vi "Flat sequence in LabVIEW.vi"() -> ()   [LabVIEW 2026]
panel:
  out "MULTIPLY":dbl
  out "MINUS":dbl
  out "SUM":dbl
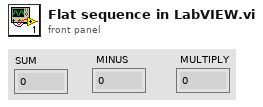
[diagram p1: front panel]
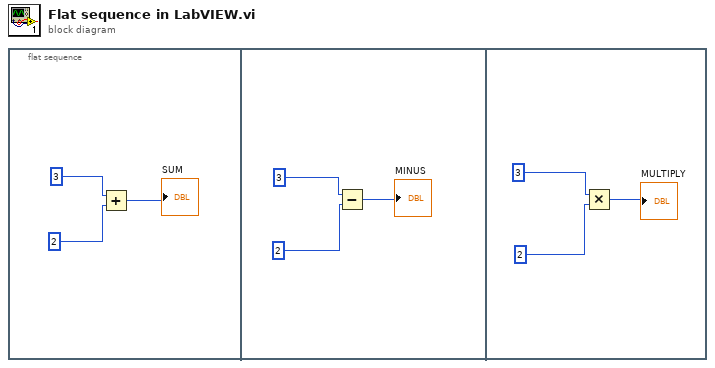
[diagram p0: block diagram]
diagram:
  n1 = flat-sequence {
    frame #0 {
      n2 = Add(x=3, y=2) -> (x+y=→"SUM":i32)
    }
    frame #1 {
      n3 = Subtract(x=3, y=2) -> (x-y=→"MINUS":i32)
    }
    frame #2 {
      n4 = Multiply(x=3, y=2) -> (x*y=→"MULTIPLY":i32)
    }
  }
